vi "Resize.vi"(10 "Capacity":u32, 11 "TypedCircularBuffer in":refnum<class "LogCircularBuffer.lvclass">) -> (3 "TypedCircularBuffer out":refnum<class "LogCircularBuffer.lvclass">)   [LabVIEW 2024, in "LogCircularBuffer.lvclass"]
uses:
  LogCircularBuffer.lvclass
  LogCircularBuffer.lvclass/LogCircularBuffer.ctl
  Type.ctl
  RQMHCore/ErrorReporting/Record/LogRecord.lvclass
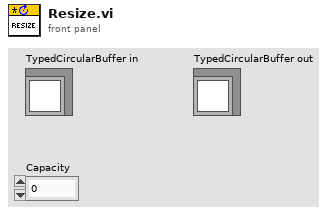
[diagram p1: front panel]
types:
  T1 = typedef "LogCircularBuffer.lvclass/Type.ctl" = refnum<class "LogRecord.lvclass">
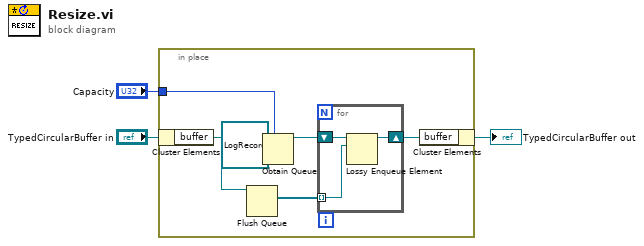
[diagram p0: block diagram]
diagram:
  n1 = in-place {
    in-place-border: "Capacity" -> [w7]
    n2 = in-place-cluster #1("TypedCircularBuffer in") -> ("buffer"=w8:refnum<queue>)
    n3 = Flush Queue(queue=w8) -> (remaining elements=w4:T1[])  [unwired: 1 in, 2 out]
    n4 = Obtain Queue(max queue size (-1, unlimited)=w7, element data type=T1 refnum ("Type")) -> (queue out=w6:refnum<queue>)  [unwired: 3 in, 2 out]
    n5 = for {
      shift-right: [w11] -> w5
      shift-left: w6 -> [w12]
      tunnel: w4 -> [w10] mode=indexing
      n6 = Lossy Enqueue Element(queue=w12, element=w10) -> (queue out=w11:refnum<queue>)  [unwired: 1 in, 3 out]
    }
    n7 = in-place-cluster #1("buffer"=w5) -> (→"TypedCircularBuffer out":refnum<class "LogCircularBuffer.lvclass">)
  }
